vi "ORS_ImgQuickRecaForConfig.vi"(0 "RecalFringePhaseFit_Inv":dbl[](array[numeric]), 1 "RecalFringePhaseFit":dbl[](array[numeric]), 2 "window parameter":dbl=nan, 3 "Offset":i32, 4 "Data input":i16[](array[numeric]), 5 "DualBackground":i16[](array[numeric]), 6 "# zeros added":i32, 7 "Sample rate":dbl=6.564640249473632 format="%#_4g", 8 "Linearization method":u16=1, 9 "subtract background plot":bool=TRUE, 11 "DLL path":path=path "FOO.dll", 12 "Window":T1=62 items=["Rectangle"=0, "Hanning"=1, "Hamming"=2, "Blackman-Harris"=3, "Exact Blackman"=4, "Blackman"=5, "Flat Top"=6, "4 Term B-Harris "=7, "7 Term B-Harris"=8, "Low Sidelobe"=9, "Blackman Nuttall"=11, "Triangle"=30, "Bartlett-Hanning"=31, "Bohman"=32, "Parzen"=33, "Welch"=34, "Kaiser"=60, "Dolph-Chebyshev"=61, "Gaussian"=62], 13 "Cursor List":T2, 14 "Cursor crop?":bool=TRUE, 16 "Use DLL":bool=TRUE, 19 "Log?":bool) -> (20 "graph output":dbl[](array[numeric]), 21 "FFT max":dbl=6.564640249473632 format="%#_4g", 24 "cursor diff sps":dbl, 25 "FFT max index":i32, 27 "FFT max freq (MHz)":dbl=6.564640249473632 format="%#_4g")   [LabVIEW 2014]
uses:
  <vilib>/Utility/miscctls.llb/LVCursorListTypeDef.ctl
  <vilib>/Analysis/4window.llb/windowTd.ctl
  <vilib>/Analysis/baseanly.llb/Mean (DBL).vi
  <vilib>/Analysis/NI_AALBase.lvlib
  <vilib>/Analysis/NI_AALPro.lvlib
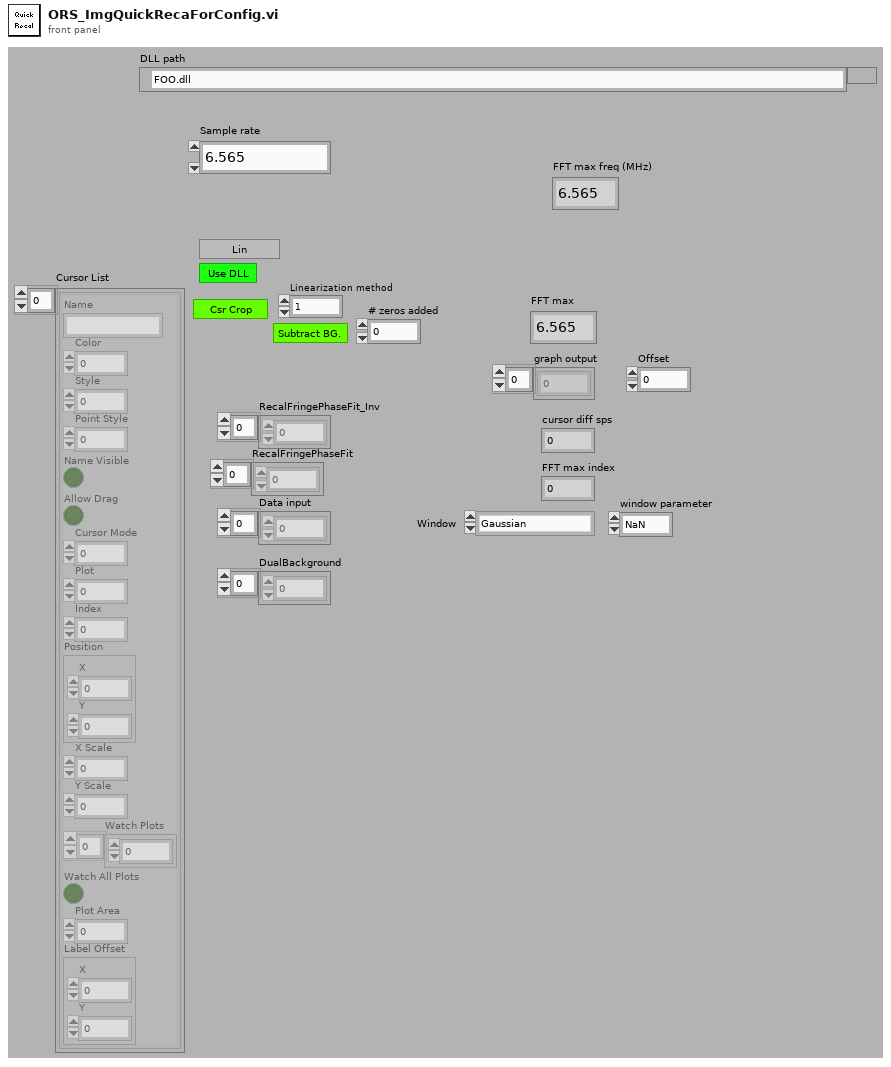
[diagram p1: front panel]
types:
  T1 = typedef "NI_AALPro.lvlib/windowTd.ctl" = u32
  T2 = typedef "LVCursorListTypeDef.ctl" = cluster{"Name":string, "Color":u32, "Style":u8, "Point Style":u8, "Name Visible":bool, "Allow Drag":bool, "Cursor Mode":u32, "Plot":i32, "Index":i32, "Position":cluster{"X":dbl, "Y":dbl}, "X Scale":u32, "Y Scale":u32, "Watch Plots":i32[], "Watch All Plots":bool, "Plot Area":i32, "Label Offset":cluster{"X":dbl, "Y":dbl}}[]
  T3 = cluster{"Name":string, "Color":u32, "Style":u8, "Point Style":u8, "Name Visible":bool, "Allow Drag":bool, "Cursor Mode":u32, "Plot":i32, "Index":i32, "Position":cluster{"X":dbl, "Y":dbl}, "X Scale":u32, "Y Scale":u32, "Watch Plots":i32[], "Watch All Plots":bool, "Plot Area":i32, "Label Offset":cluster{"X":dbl, "Y":dbl}}
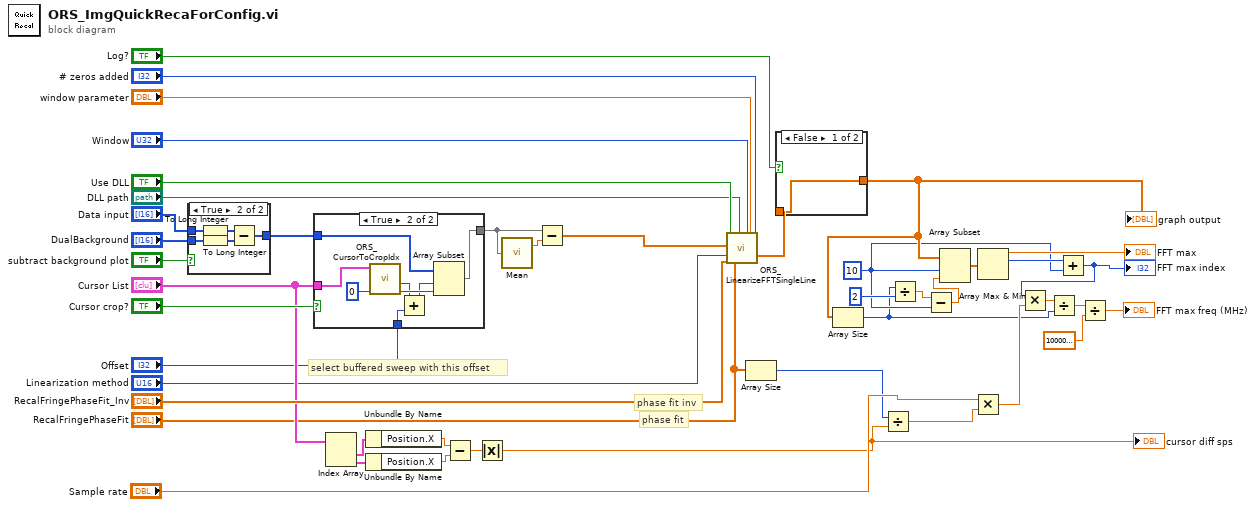
[diagram p0: block diagram]
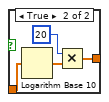
[diagram p2: hidden frame]
diagram:
  w17 = 10 ("index")
  # "select buffered sweep with this offset"
  # "phase fit"
  # "phase fit inv"
  n1 = case shown="True" "subtract background plot" {
    tunnel: "DualBackground" -> [_ w49]
    tunnel: [w45 w50] -> w40
    tunnel: "Data input" -> [w45 w48]
    frame False {
    }
    frame True {
      n2 = To Long Integer(number=w48) -> (32bit integer=w47:i32[])
      n3 = To Long Integer(number=w49) -> (32bit integer=w46:i32[])
      n4 = Subtract(x=w47, y=w46) -> (x-y=w50:i32[])
    }
  }
  n5 = case shown="True" "Cursor crop?" {
    tunnel: [w51 w57] -> w42
    tunnel: w40 -> [w51 w56]
    tunnel: "Cursor List" -> [_ w55]
    tunnel: "Offset" -> [_ w52]
    frame False {
    }
    frame True {
      n6 = call "ORS_CursorToCropIdx.vi"("index offset"=0 ("index 1"), "Cursor List"=w55) -> ("length"=w59:i32, "offset"=w54:i32)  [unwired: 8 in]
      n7 = Add(x=w54, y=w52) -> (x+y=w53:i32)
      n8 = Array Subset(array=w56, index=w53, length=w59) -> (w57:i32[])
    }
  }
  n9 = Index Array(array="Cursor List") -> (element #1=w33:T3, element #2=w32:T3)  [unwired: 2 in]
  n10 = Unbundle By Name(w33) -> ("Position.X"=w30:dbl)
  n11 = Unbundle By Name(w32) -> ("Position.X"=w31:dbl)
  n12 = Subtract(x=w30, y=w31) -> (x-y=w29:dbl)
  n13 = Absolute Value(x=w29) -> (abs(x)=w10:dbl)
  "cursor diff sps" <- w10
  n14 = call-poly <vilib>:"Mean.vi"("X"=w42) -> ("mean"=w44:dbl)  [unwired: 1 out]
  n15 = Subtract(x=w42, y=w44) -> (x-y=w7:dbl[])
  n16 = call "ORS_LinearizeFFTSingleLine.vi"("Michelson fringes"=w7, "Linearization method"="Linearization method", "inverted Hilbert in"="RecalFringePhaseFit_Inv", "Use DLL"="Use DLL", "RecalFringePhaseFit"="RecalFringePhaseFit", "DLL path"="DLL path", "Window"="Window", "window parameter"="window parameter", "# zeros added"="# zeros added") -> ("Output"=w41:dbl[])  [unwired: 10 in]
  n17 = Array Size(array="RecalFringePhaseFit") -> (size(s)=w9:i32)
  n18 = case shown="False" "Log?" {
    tunnel: w41 -> [w60 w64]
    tunnel: [w60 w61] -> w25
    frame False {
    }
    frame True {
      n19 = Logarithm Base 10(1:w64) -> (0:w63:dbl[])
      n20 = Multiply(x=20 ("index 1"), y=w63) -> (x*y=w61:dbl[])
    }
  }
  "graph output" <- w25
  n21 = Array Size(array=w25) -> (size(s)=w12:i32)
  n22 = Divide(x=w9, y=w10) -> (x/y=w13:dbl)
  n23 = Divide(x=w12, y=2 ("index")) -> (x/y=w23:dbl)
  n24 = Subtract(x=w23, y=w17) -> (x-y=w24:dbl)
  n25 = Array Subset(array=w25, index=w17, length=w24) -> (w26:dbl[])
  n26 = Multiply(x="Sample rate", y=w13) -> (x*y=w15:dbl)
  n27 = Array Max & Min(array=w26) -> (max value=→"FFT max":dbl, max index (indices)=w18:i32)  [unwired: 2 out]
  n28 = Add(x=w18, y=w17) -> (x+y=w16:i32)
  "FFT max index" <- w16
  n29 = Multiply(x=w16, y=w15) -> (x*y=w27:dbl)
  n30 = Divide(x=w27, y=w12) -> (x/y=w21:dbl)
  n31 = Divide(x=w21, y=1000000.0) -> (x/y=→"FFT max freq (MHz)":dbl)
